vi "file_read_binary_pkt.vi"(8 "error in (no error)":errorcluster, 9 "Packet No.":i32, 10 "Pkt Size(bytes)":i32, 11 "Byte Stream File in":refnum<file>) -> (0 "error out":errorcluster, 1 "EOF?":bool, 2 "Packet":string, 3 "Byte Stream File out":refnum<file>)   [LabVIEW 2018]
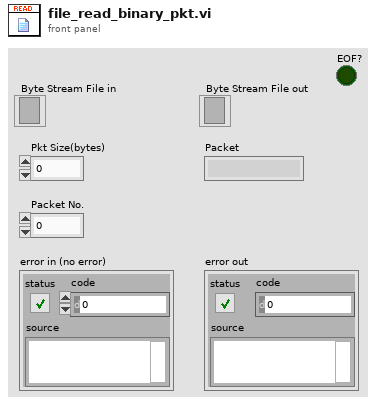
[diagram p1: front panel]
types:
  T1 = enum16{"big-endian, network order", "native, host order", "little-endian"}
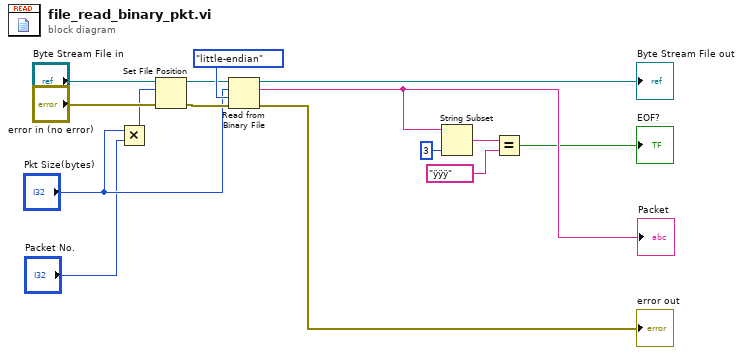
[diagram p0: block diagram]
diagram:
  n1 = Multiply(x="Pkt Size(bytes)", y="Packet No.") -> (x*y=w8:i32)
  n2 = Set File Position(offset (in bytes) (0)=w8, refnum="Byte Stream File in") -> (refnum out=w13:refnum<file>)  [unwired: 2 in, 1 out]
  n3 = Read from Binary File(8:"error in (no error)", 9:T1."little-endian" ("byte order (0:big-endian, network order)"), 10:"Pkt Size(bytes)", 11:w13) -> (0:→"error out":errorcluster, 2:w5:string, 3:→"Byte Stream File out":refnum<file>)  [unwired: 2 in, 1 out]
  "Packet" <- w5
  n4 = String Subset(string=w5, length (rest)=3 ("length (rest)")) -> (substring=w3:string)  [unwired: 1 in]
  n5 = Equal?(x=w3, y="ÿÿÿ") -> (x = y?=→"EOF?":bool)
